vi "NthDerivativeOfScalarVariable.vi"(8 "Reset?":bool, 9 "Derivative level":i32=1 min=-10 max=10, 10 "FPGA Timestamp":dbl, 11 "X":dbl) -> (3 "Nth derivative of X":dbl)   [LabVIEW 2014]
doc: "This VI is designed to take the Nth derivative (negative N values indicate integration) without requiring the history of X, i.e, reading an analog value in a loop, and taking the Nth derivative at the current time."
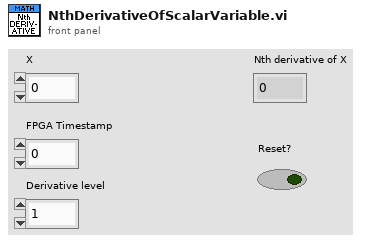
[diagram p1: front panel]
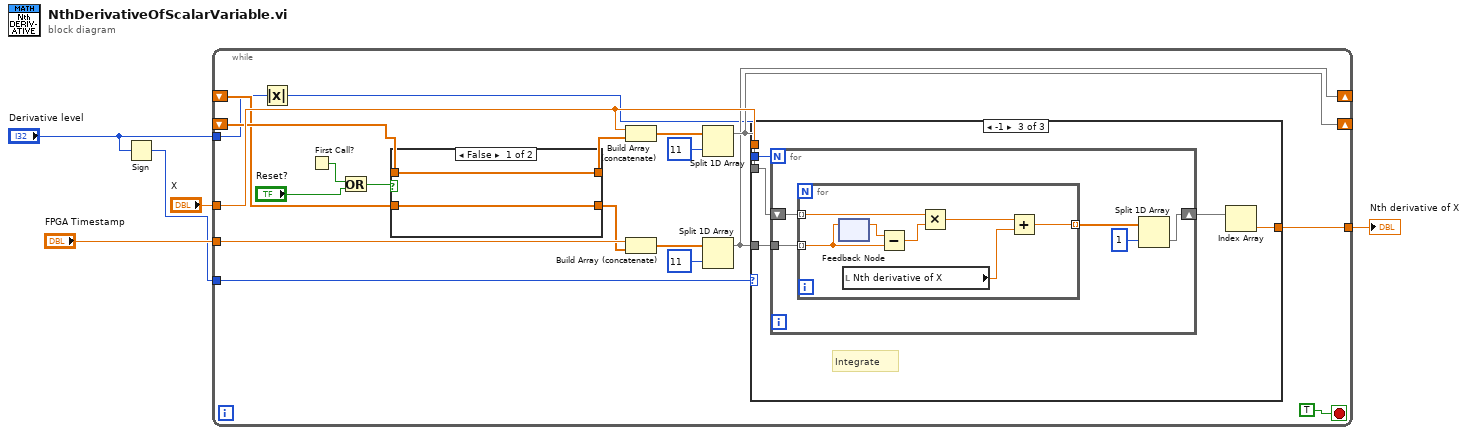
[diagram p0: block diagram]
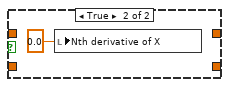
[diagram p2: hidden frame]
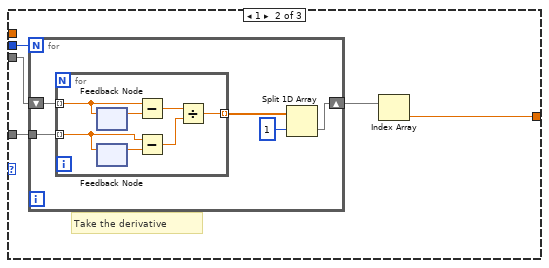
[diagram p4: hidden frame]
diagram:
  n1 = Sign(1:"Derivative level") -> (0:w3:i32)
  n2 = while {
    tunnel: "X" -> [w18]
    shift-right: [w11] -> _
    shift-left: _ -> [w14]
    tunnel: "FPGA Timestamp" -> [w23]
    shift-right: [w12] -> _
    shift-left: _ -> [w16]
    tunnel: w3 -> [w19]
    tunnel: [w17] -> w2
    tunnel: "Derivative level" -> [w10]
    stop <- TRUE stop-if-true
    n3 = Absolute Value(x=w10) -> (abs(x)=w9:i32)
    n4 = First Call?() -> (First Call?: T/F=w6:bool)
    n5 = Or(x=w6, y="Reset?") -> (x .or. y?=w8:bool)
    n6 = case shown="False" w8 {
      tunnel: w16 -> [w27 _]
      tunnel: [w27 _] -> w15
      tunnel: w14 -> [w26 _]
      tunnel: [w26 _] -> w13
      frame False {
      }
      frame True {
        n7 = local write "Nth derivative of X"(0.0 ("Nth derivative of X")) -> ()
      }
    }
    n8 = Build Array (concatenate)(w18, w15) -> (w25:dbl[])
    n9 = Build Array (concatenate)(w23, w13) -> (w21:dbl[])
    n10 = Split 1D Array(array=w25, index=11) -> (first subarray=w12:dbl[])  [unwired: 1 out]
    n11 = Split 1D Array(array=w21, index=11) -> (first subarray=w11:dbl[])  [unwired: 1 out]
    n12 = case shown="-1" w19 {
      tunnel: w18 -> [w29 _ _]
      tunnel: [w29 w31 w48] -> w17
      tunnel: w9 -> [_ w34 w51]
      tunnel: w11 -> [_ w32 w49]
      tunnel: w12 -> [_ w33 w50]
      frame 0, Default {
        # "0th derivative, don't change X"
      }
      frame 1 {
        # "Take the derivative"
        n13 = for {
          N: w34 -> [_]
          shift-right: [w35] -> w30
          shift-left: w33 -> [w39]
          tunnel: w32 -> [w38]
          n14 = for {
            tunnel: w39 -> [w46] mode=indexing
            tunnel: w38 -> [w43] mode=indexing
            tunnel: [w40] -> w37 mode=indexing
            n15 = feedback-in #1(w46) -> ()
            n16 = feedback #1() -> (w45:dbl)  [unwired: 1 in]
            n17 = feedback #2() -> (w44:dbl)  [unwired: 1 in]
            n18 = feedback-in #2(w43) -> ()
            n19 = Subtract(x=w46, y=w45) -> (x-y=w41:dbl)
            n20 = Subtract(x=w43, y=w44) -> (x-y=w42:dbl)
            n21 = Divide(x=w41, y=w42) -> (x/y=w40:dbl)
          }
          n22 = Split 1D Array(array=w37, index=1) -> (second subarray=w35:dbl[])  [unwired: 1 out]
        }
        n23 = Index Array(array=w30) -> (element=w31:dbl)  [unwired: 1 in]
      }
      frame -1 {
        # "Integrate"
        n24 = for {
          N: w51 -> [_]
          shift-right: [w52] -> w47
          shift-left: w50 -> [w56]
          tunnel: w49 -> [w55]
          n25 = for {
            tunnel: w56 -> [w62] mode=indexing
            tunnel: w55 -> [w57] mode=indexing
            tunnel: [w61] -> w54 mode=indexing
            n26 = feedback #3() -> (w58:dbl)  [unwired: 1 in]
            n27 = feedback-in #3(w57) -> ()
            n28 = local read "Nth derivative of X"() -> (w59:dbl)
            n29 = Subtract(x=w58, y=w57) -> (x-y=w63:dbl)
            n30 = Multiply(x=w62, y=w63) -> (x*y=w60:dbl)
            n31 = Add(x=w60, y=w59) -> (x+y=w61:dbl)
          }
          n32 = Split 1D Array(array=w54, index=1) -> (second subarray=w52:dbl[])  [unwired: 1 out]
        }
        n33 = Index Array(array=w47) -> (element=w48:dbl)  [unwired: 1 in]
      }
    }
  }
  "Nth derivative of X" <- w2
